vi "LithographyPointsSendToIgor.vi"(8 "error in (no error)":errorcluster, 10 "Interpolation":i32, 11 "Asylum_Driver in":refnum<class "Asylum_Driver.lvclass">) -> (0 "error out":errorcluster, 2 "TempFileNames":path[](array[path]), 3 "Asylum_Driver out":refnum<class "Asylum_Driver.lvclass">)   [LabVIEW 2019, in "Asylum_Driver.lvclass"]
uses:
  Asylum_Driver.lvclass
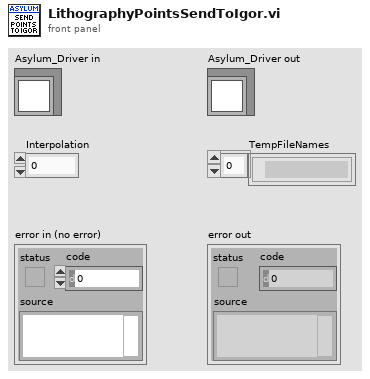
[diagram p1: front panel]
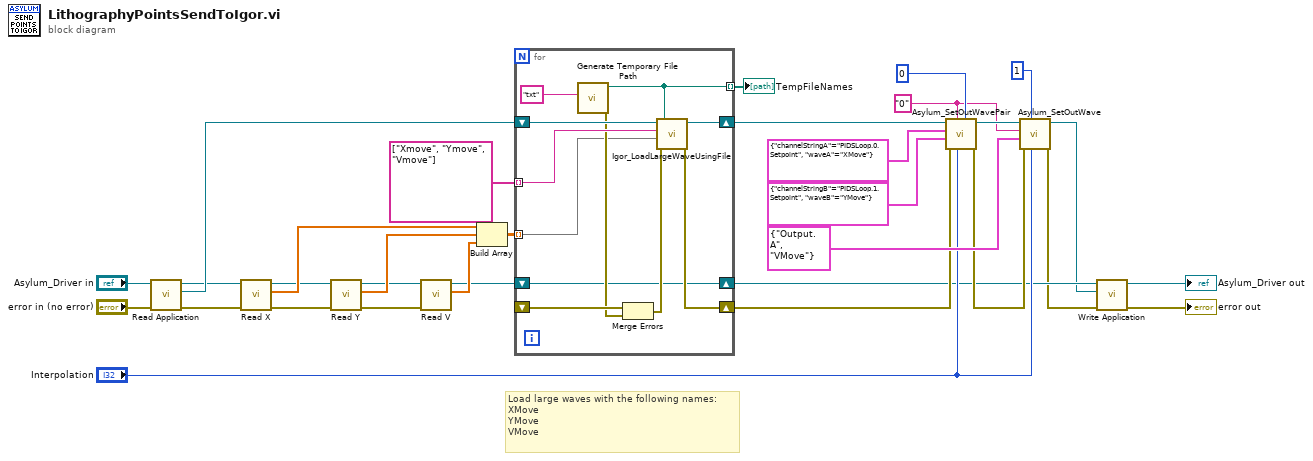
[diagram p0: block diagram]
diagram:
  w26 = "0" ("eventString")
  # "Load large waves with the following names:\nXMove\nYMove\nVMove"
  n1 = call-dynamic "Read Application.vi"("Asylum_Driver in"="Asylum_Driver in") -> ("Application"=w16:refnum<k7>, "Asylum_Driver out"=w11:refnum<class "Asylum_Driver.lvclass">)  [unwired: 9 in]
  n2 = call-dynamic "Read X.vi"("error in (no error)"="error in (no error)", "Asylum_Driver in"=w11) -> ("error out"=w6:errorcluster, "X"=w15:dbl[], "Asylum_Driver out"=w10:refnum<class "Asylum_Driver.lvclass">)  [unwired: 7 in]
  n3 = call-dynamic "Read Y.vi"("error in (no error)"=w6, "Asylum_Driver in"=w10) -> ("error out"=w5:errorcluster, "Y"=w14:dbl[], "Asylum_Driver out"=w9:refnum<class "Asylum_Driver.lvclass">)  [unwired: 7 in]
  n4 = call-dynamic "Read V.vi"("error in (no error)"=w5, "Asylum_Driver in"=w9) -> ("V"=w13:dbl[], "Asylum_Driver out"=w8:refnum<class "Asylum_Driver.lvclass">)  [unwired: 7 in, 1 out]
  n5 = Build Array(w15, w14, w13) -> (w19:dbl[][])
  n6 = for {
    tunnel: w19 -> [w32] mode=indexing
    shift-right: [w41] -> w21
    shift-left: _ -> [w35]
    tunnel: string[] ["Xmove", "Ymove", "Vmove"] -> [w39] mode=indexing
    shift-right: [w38] -> w25
    shift-left: w16 -> [w40]
    tunnel: [w36] -> w3 mode=indexing
    shift-right: [w31] -> w7
    shift-left: w8 -> [w31]
    n7 = call <vilib>:"Generate Temporary File Path.vi"("Temporary File Extension (tmp)"="txt") -> ("error out"=w34:errorcluster, "Unique Temporary File Path"=w36:path)  [unwired: 9 in]
    n8 = Merge Errors(w35, w34) -> (w33:errorcluster)
    n9 = call <userlib>:"Igor_LoadLargeWaveUsingFile.vi"("Path"=w36, "error in"=w33, "Wave"=w32, "Wavename"=w39, "Application"=w40) -> ("error out"=w41:errorcluster, "Application"=w38:refnum<k7>)  [unwired: 5 in]
  }
  "TempFileNames" <- w3
  n10 = call <userlib>:"Asylum_SetOutWavePair.vi"("whichBank"=0, "interpolation"="Interpolation", "eventString"=w26, "error in (no error)"=w21, "Wave B"=cluster{"channelStringB":string, "waveB":string} {"channelStringB"="PIDSLoop.1.Setpoint", "waveB"="YMove"}, "Wave A"=cluster{"channelStringA":string, "waveA":string} {"channelStringA"="PIDSLoop.0.Setpoint", "waveA"="XMove"}, "Application"=w25) -> ("error out"=w23:errorcluster, "Application"=w27:refnum<k7>)  [unwired: 3 in]
  n11 = call <userlib>:"Asylum_SetOutWave.vi"("interpolation"="Interpolation", "whichBank"=1, "error in (no error)"=w23, "Wave"=cluster{"channelString":string, "wave":string} {"channelString"="Output.A", "wave"="VMove"}, "eventString"=w26, "Application"=w27) -> ("error out"=→"error out":errorcluster, "Application"=w4:refnum<k7>)  [unwired: 4 in]
  n12 = call-dynamic "Write Application.vi"("Application"=w4, "Asylum_Driver in"=w7) -> ("Asylum_Driver out"=→"Asylum_Driver out":refnum<class "Asylum_Driver.lvclass">)  [unwired: 9 in]
